vi "SENS_CORR_CSET_SAVE.vi"(0 "VISA IN":refnum<visa-resource-name>, 1 "USER01...10":string, 5 "error in":errorcluster, 7 "Channel":i32) -> (14 "VISA Out":refnum<visa-resource-name>, 19 "error out":errorcluster)   [LabVIEW 2018, in "PNA-X.lvlib"]
doc: "SENSe<cnum>:CORRection:CSET:SAVE <char> \n1696\n\nThis command is NOT necessary after completion of a calibration. A Cal Set is automatically created, \napplied to the channel, and saved at the completion of a guided cal according to the preference setting \nSENS:CORR:PREF:CSET:SAVE. \n(Read Write) \nSaves the channel's Cal Set to the PNA hard drive. For example, use this command after writing data \nto a Cal Set using SENS:CORR:CSET:DATA (For Advanced Users). \nThe file name is saved as \"CSETx.cst\" where x is the user number assigned to <char>, and .cst \nspecifies a Cal Set and instrument state. This is not the same syntax as a file saved through the default \nchoices from the front panel, which is \"at00x.cst\". For more information on the file naming syntax, \nsee the MMEMory subsystem. Learn more about Instrument/Cal States. \nParameters \n<cnum> Any existing channel number. If unspecified, value is set to 1 \n<char> Choose from: \nUSER01 \nUSER02... \nUSER10 \nExamples SENS:CORR:CSET:SAVE USER03 \nsense2:correction:cset:save user09 \nQuery Syntax SENSe<cnum>:CORRection:CSET:SAVE? \nQueries the last correction set saved. \nReturn Type Character \nDefault Not applicable \nSENSe:CORRection:CSET:TSET:ALLPorts? <cset> \n1697\n\n(Read-only) Reads the port mapping used for the specified Cal Set. The returned values are the \nphysical ports. The POSITION of the returned values corresponds to the logical ports. \nFor example, with an N44xx test set, if the returned string is \"PNA 1,TS 2,PNA 2, TS 4\" this means: \nPNA 1 is assigned to logical port 1 \nTS 2 is assigned to logical port 2 \nPNA 2 is assigned to logical port 3 \nTS 4 is assigned to logical port 4 \nParameters \n<cset> (String) Name or GUID of the Cal Set. Use SENS:CORR:CSET:CAT? to read \nthe list of available Cal Set names or GUIDs. \nExamples SENS:CORR:CSET:TSET:ALLP? \"MyCalSet\" \nsens:correction:cset:tset:allports? \"{2B893E7A-971A-11d5-8D6C- \n00108334AE96}\" \nReturn Type String \nDefault Not Applicable \nSENSe:CORRection:CSET:TSET:TYPE? <cset> \n(Read-only) Reads the test set type (model) used for the specified Cal Set. \nParameters \n<cset> (String) Name or GUID of the Cal Set. Use SENS:CORR:CSET:CAT? to read \nthe list of available Cal Set names or GUIDs. \nExamples SENS:CORR:CSET:TSET:TYPE? \"MyCalSet\" \n'returns \"N44xx\" \nsens:correction:cset:tset:type? \"{2B893E7A-971A-11d5-8D6C- \n00108334AE96}\" \nReturn Type String \nDefault Not Applicable \nSENSe<ch>:CORRection:CSET:TYPE:CATalog? [format] \n1698\n\n(Read-only) Query the Cal Types available in the selected Cal Set. The output is a comma separated \nlist of Guids or a Cal Type names. Learn more about applying Cal Types using SCPI. \nUse CALC:CORR:TYPE to apply a Cal Type. \nParameters \n<ch> Any existing channel number. If unspecified, value is set to 1 \n[format] (Optional) Format of the output of cal types. choose from: \nNAME - (default) returns a list of cal type string names. \nGUID - returns a list of cal type GUIDs \nExamples SENS:CORR:CSET:TYPE:CAT? NAME \nSENS2:CORRection:CSET:TYPE:CAT? \nReturn Type String \nDefault Not Applicable \nLast modified: \n9/12/06 MQ Added TSET commands for multiport. \n1699\n\nSense:Correction:Extension Commands \nPerforms and applies Port Extensions. \nClick on a blue keyword to view the command details. \nSee Also \nExample Programs \nLearn about Port Extensions \nSynchronizing the PNA and Controller \nSCPI Command Tree"
uses:
  PNA-X.lvlib
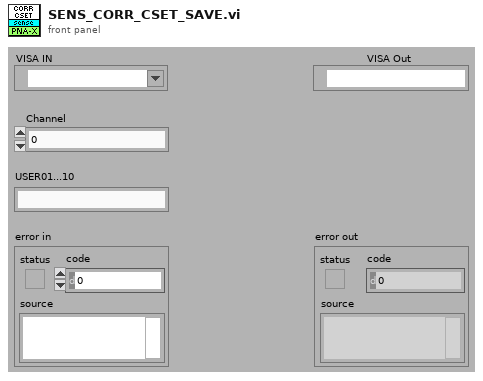
[diagram p1: front panel]
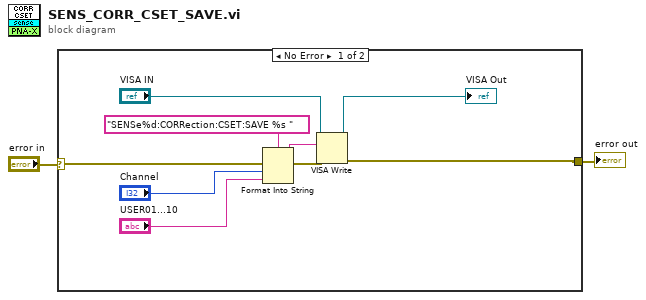
[diagram p0: block diagram]
diagram:
  n1 = case shown="No Error" "error in" {
    selector: "error in" -> [w11 w12]
    tunnel: [w6 w12] -> w1
    frame No Error {
      n2 = Format Into String(format string="SENSe%d:CORRection:CSET:SAVE %s " ("Cmdline"), error in=w11, "Channel", "USER01...10") -> (resulting string=w9:string, error out=w10:errorcluster)  [unwired: 1 in]
      n3 = VISA Write(VISA resource name="VISA IN", write buffer=w9, error in (no error)=w10) -> (VISA resource name out=→"VISA Out":refnum<visa-resource-name>, error out=w6:errorcluster)  [unwired: 1 out]
    }
    frame Error {
    }
  }
  "error out" <- w1
